vi "Read Diode.vi"(8 "error in (no error)":errorcluster, 11 "Fluke DMM in":refnum<class "Fluke DMM.lvclass">) -> (0 "error out":errorcluster, 2 "Diode Voltage":dbl, 3 "Fluke DMM out":refnum<class "Fluke DMM.lvclass">)   [LabVIEW 2011, in "Fluke DMM.lvclass"]
uses:
  Fluke DMM.lvclass
  Fluke DMM.lvclass/Fluke DMM.ctl
  <instrlib>/Fluke 884X Series/Public/Data/Read (Single Point).vi
  <instrlib>/Fluke 884X Series/Fluke 884X Series.lvlib
panel:
  in  "Function (0: DC Voltage)":u16(ring)=9 items=["DC Voltage", "AC Voltage", "2 - Wire Resistance", "4 - Wire Resistance", "DC Current", "AC Current", "Frequency", "Period", "Continuity", "Diode Checking", "Temperature", "Capacitance"]
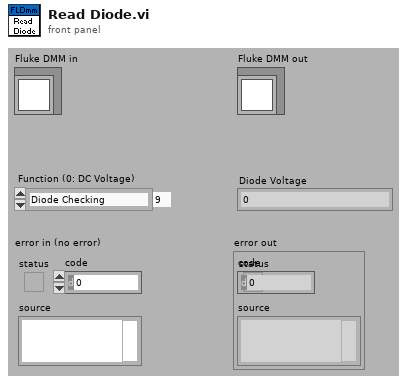
[diagram p1: front panel]
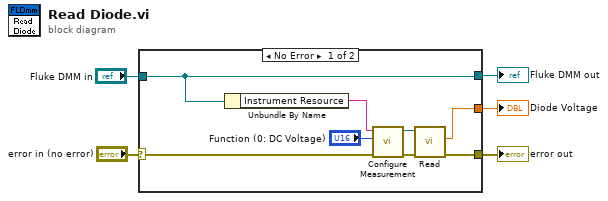
[diagram p0: block diagram]
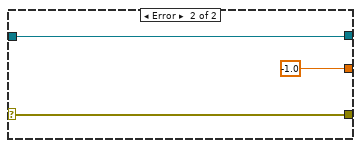
[diagram p2: hidden frame]
diagram:
  n1 = case shown="No Error" "error in (no error)" {
    selector: "error in (no error)" -> [w8 w16]
    tunnel: [w10 w16] -> w4
    tunnel: [w9 -1.0 ("Measurement Data")] -> w1
    tunnel: "Fluke DMM in" -> [w7 w14]
    tunnel: [w7 w14] -> w2
    frame No Error {
      n2 = Unbundle By Name(w7) -> ("Instrument Resource"=w6:string)
      n3 = call <instrlib>:"Configure Measurement.vi"("error in (no error)"=w8, "Function (0: DC Voltage)"="Function (0: DC Voltage)", "VISA resource name"=w6) -> ("error out"=w11:errorcluster, "VISA resource name out"=w12:refnum<visa-resource-name>)  [unwired: 3 in, 4 out]
      n4 = call-poly <instrlib>:"Read.vi"("error in (no error)"=w11, "VISA resource name"=w12) -> ("error out"=w10:errorcluster, "Measurement"=w9:dbl)  [unwired: 8 out]
    }
    frame Error {
    }
  }
  "error out" <- w4
  "Fluke DMM out" <- w2
  "Diode Voltage" <- w1
